vi "json_decode_string.vi"(8 "error in (no error)":errorcluster, 11 "json":string) -> (0 "error out":errorcluster, 2 "remaining json":string, 3 "value":variant)   [LabVIEW 2017, in "rethinkdb.lvlib"]
uses:
  rethinkdb.lvlib
  <vilib>/regexp/Match Regular Expression.xnode
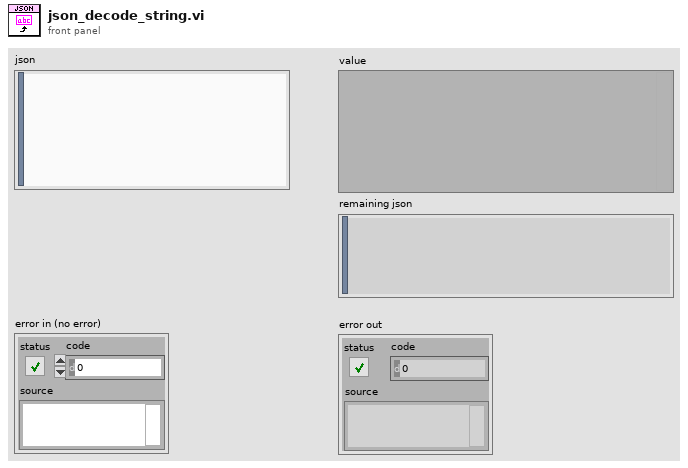
[diagram p1: front panel]
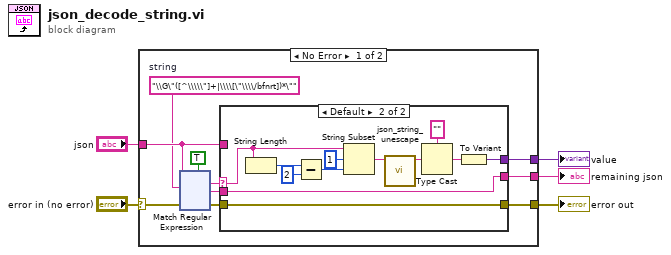
[diagram p0: block diagram]
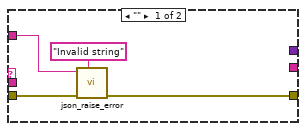
[diagram p2: hidden frame]
diagram:
  n1 = case shown="No Error" "error in (no error)" {
    selector: "error in (no error)" -> [w7 w146]
    tunnel: "json" -> [w12 _]
    tunnel: [w15 w146] -> w4
    tunnel: [w14 _] -> w2
    tunnel: [w9 _] -> w1
    frame No Error {
      w11 = "\\G\"([^\\\\\"]+|\\\\[\"\\\\/bfnrt])*\""  # string
      n2 = xnode "Match Regular Expression"("input string"=w12, "regular expression"=w11, "error in"=w7, "multiline? (F)"=TRUE) -> ("whole match"=w13:string, "after match"=w8:string, "error out"=w6:errorcluster)  [unwired: 2 in, 2 out]
      n3 = case shown="Default" w13 {
        selector: w13 -> [_ w136]
        tunnel: [w131 w144] -> w15
        tunnel: w6 -> [w133 w144]
        tunnel: [_ w145] -> w14
        tunnel: w12 -> [w132 _]
        tunnel: [_ w134] -> w9
        tunnel: w8 -> [_ w134]
        frame "" {
          n4 = call "json_raise_error.vi"("message"="Invalid string" ("error message (\"\")"), "error in (no error)"=w133, "json"=w132) -> ("error out"=w131:errorcluster)  [unwired: 8 in]
        }
        frame Default {
          n5 = String Length(string=w136) -> (length=w135:i32)
          n6 = Subtract(x=w135, y=2) -> (x-y=w140:i32)
          n7 = String Subset(string=w136, offset (0)=1, length (rest)=w140) -> (substring=w143:string)
          n8 = call "json_string_unescape.vi"("escaped string"=w143) -> ("string out"=w139:string)  [unwired: 9 in, 1 out]
          n9 = Type Cast(type="", x=w139) -> (*(type *) &x=w138:string)
          n10 = To Variant(anything=w138) -> (Variant=w145:variant)
        }
      }
    }
    frame Error {
    }
  }
  "error out" <- w4
  "value" <- w2
  "remaining json" <- w1
